vi "LockUnlockResultManager.vi"(8 "semaphore (optional)":T1, 11 "Lock? (T)":bool=TRUE) -> (0 "semaphore":T1, 2 "Valid non-zero instance":bool, 3 "ResultManager":T2)   [LabVIEW 2011]
uses:
  qtrk/QTrkLVBinding/ResultManagerInstance.ctl
  SemaphoreResultManager.vi
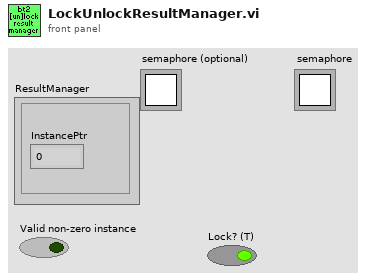
[diagram p1: front panel]
types:
  T1 = typedef "Semaphore RefNum" = refnum<k1>
  T2 = typedef "ResultManagerInstance.ctl" = cluster{"InstancePtr":u64}
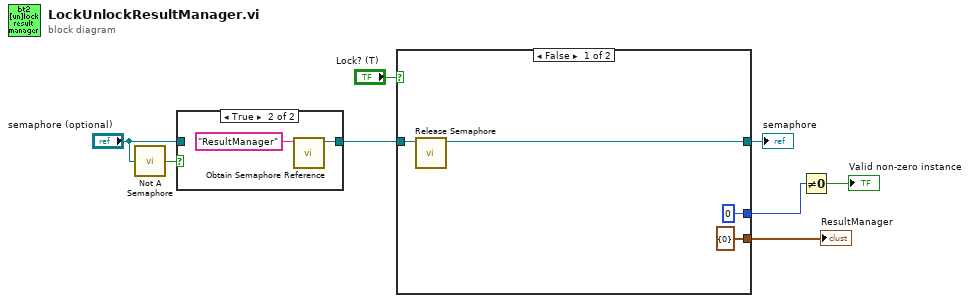
[diagram p0: block diagram]
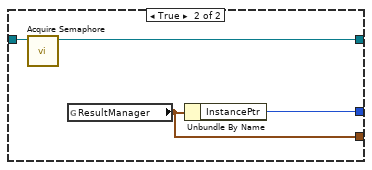
[diagram p3: hidden frame]
diagram:
  n1 = call <vilib>:"Not A Semaphore.vi"("semaphore"="semaphore (optional)") -> ("not a semaphore"=w5:bool)
  n2 = case shown="True" w5 {
    tunnel: [w9 w10] -> w4
    tunnel: "semaphore (optional)" -> [w9 _]
    frame False {
    }
    frame True {
      n3 = call <vilib>:"Obtain Semaphore Reference.vi"("name (unnamed)"="ResultManager") -> ("semaphore"=w10:T1)  [unwired: 4 in, 2 out]
    }
  }
  n4 = case shown="False" "Lock? (T)" {
    tunnel: w4 -> [w15 w19]
    tunnel: [w14 w18] -> w6
    tunnel: [cluster{"InstancePtr":u64} {"InstancePtr"=0} ("ResultManager") w17] -> w2
    tunnel: [u64 0 ("InstancePtr") w16] -> w1
    frame False {
      n5 = call <vilib>:"Release Semaphore.vi"("semaphore"=w15) -> ("semaphore out"=w14:T1)  [unwired: 5 in, 1 out]
    }
    frame True {
      n6 = call <vilib>:"Acquire Semaphore.vi"("semaphore"=w19) -> ("semaphore out"=w18:T1)  [unwired: 4 in, 2 out]
      n7 = global read "SemaphoreResultManager.vi" "ResultManager"() -> (w17:cluster{"InstancePtr":u64})
      n8 = Unbundle By Name(w17) -> ("InstancePtr"=w16:u64)
    }
  }
  "ResultManager" <- w2
  "semaphore" <- w6
  n9 = Not Equal To 0?(x=w1) -> (x != 0?=→"Valid non-zero instance":bool)
